vi "SimulateNoise.vi"(10 "Waveforms":waveform(dbl)[](array[waveform])) -> (2 "Waveforms + noise":waveform(dbl)[](array[waveform]))   [LabVIEW 2016, in "lockin.lvclass"]
uses:
  lockin.lvclass
  <vilib>/measure/NI_MABase.lvlib
  DSP.lockin/DSP_lockin.lvclass
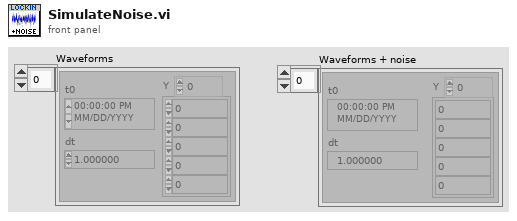
[diagram p1: front panel]
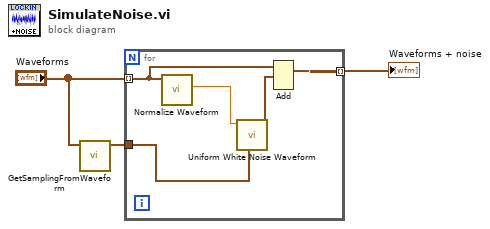
[diagram p0: block diagram]
diagram:
  n1 = call "GetSamplingFromWaveform.vi"("Waveforms"="Waveforms") -> ("sampling info"=w1:cluster{"Fs":dbl, "#s":dbl})  [unwired: 10 in]
  n2 = for {
    tunnel: "Waveforms" -> [w5] mode=indexing
    tunnel: [w7] -> w3 mode=indexing
    tunnel: w1 -> [w4]
    n3 = call <vilib>:"Normalize Waveform.vi"("waveform in"=w5) -> ("scale"=w6:dbl)  [unwired: 7 in, 3 out]
    n4 = call <vilib>:"Uniform White Noise Waveform.vi"("sampling info"=w4, "amplitude"=w6) -> ("signal out"=w8:waveform(dbl))  [unwired: 8 in, 1 out]
    n5 = Add(1:w8, 2:w5) -> (0:w7:waveform(dbl))  [unwired: 1 in, 1 out]
  }
  "Waveforms + noise" <- w3
